vi "MovingAverageZeroPhase.vi"(1 "Enable (T)":bool=TRUE, 2 "filter length (use odd number)":i32, 3 "raw array in":dbl[](array[numeric])) -> (0 "filtered array out":dbl[](array[numeric]))   [LabVIEW 2013, in "main.lvlib"]
uses:
  main.lvlib
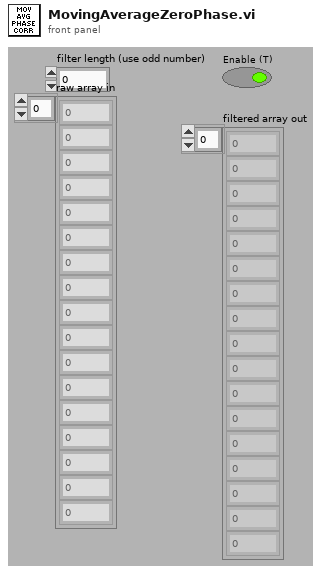
[diagram p1: front panel]
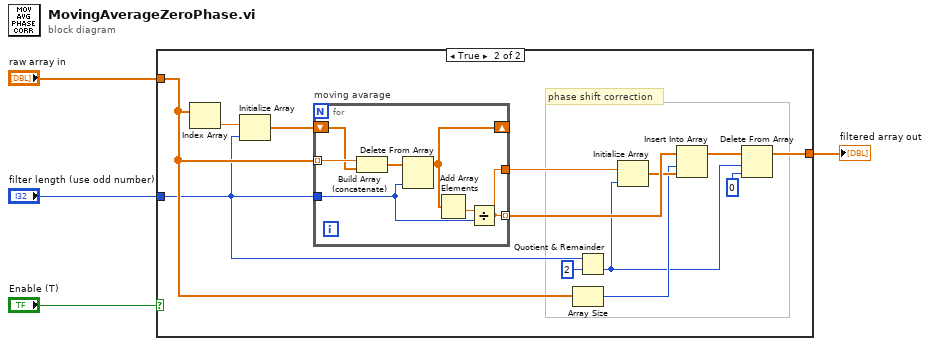
[diagram p0: block diagram]
diagram:
  n1 = case shown="True" "Enable (T)" {
    tunnel: "raw array in" -> [w5 w14]
    tunnel: "filter length (use odd number)" -> [_ w13]
    tunnel: [w5 w6] -> w2
    frame False {
    }
    frame True {
      # "phase shift correction"
      n2 = Index Array(array=w14) -> (element=w18:dbl)  [unwired: 1 in]
      n3 = Initialize Array(w18, w13) -> (w17:dbl[])
      n4 = for "moving avarage" {
        tunnel: w14 -> [w25] mode=indexing
        shift-right: [w20] -> _
        shift-left: w17 -> [w24]
        tunnel: w13 -> [w21]
        tunnel: [w19] -> w12 mode=indexing
        tunnel: [w19] -> w16
        n5 = Build Array (concatenate)(w25, w24) -> (w23:dbl[])
        n6 = Delete From Array(array=w23, index=w21) -> (array with subset deleted=w20:dbl[])  [unwired: 1 in, 1 out]
        n7 = Add Array Elements(numeric array=w20) -> (sum=w22:dbl)
        n8 = Divide(x=w22, y=w21) -> (x/y=w19:dbl)
      }
      n9 = Array Size(array=w14) -> (size(s)=w10:i32)
      n10 = Quotient & Remainder(x=w13, y=2) -> (floor(x/y)=w8:i32)  [unwired: 1 out]
      n11 = Initialize Array(w16, w8) -> (w11:dbl[])
      n12 = Insert Into Array(array=w12, index=w10, new element=w11) -> (w9:dbl[])
      n13 = Delete From Array(array=w9, length=w8, index=0) -> (array with subset deleted=w6:dbl[])  [unwired: 1 out]
    }
  }
  "filtered array out" <- w2
